vi "drag Markers.vi"(5 "Marker Options":T3={"Color"=16723218, "pen"={"Width"=2, "Style"=enum."Solid"}, "font"={"Font Name"="Arial", "Size"=16, "Strikeout?"=FALSE, "Italic?"=FALSE, "Underline?"=FALSE, "Outline?"=FALSE, "Shadow?"=FALSE, "Bold?"=FALSE, "FontColor"=0}, "caption"=""}, 7 "Type":T2, 10 "Coords":T4, 11 "Plot Area Bounds":T1) -> (3 "new picture":picture)   [LabVIEW 2019]
doc: "Draw notes overlayed on the grph using picture control elements in the graph. This draws a line at the mouse location."
uses:
  <vilib>/Utility/miscctls.llb/LVPoint32TypeDef.ctl
  controls/MarkerOptions.ctl
  controls/markerType.ctl
  <vilib>/Utility/miscctls.llb/LVRectTypeDef.ctl
panel:
  in  "picture":picture
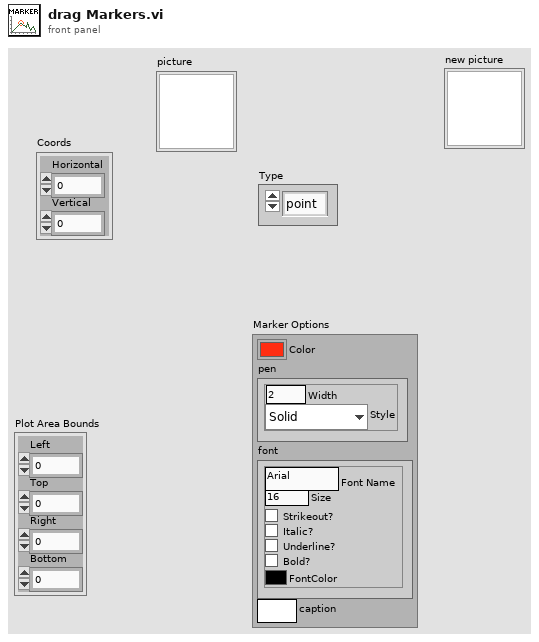
[diagram p1: front panel]
types:
  T1 = typedef "LVRectTypeDef.ctl" = cluster{"Left":i16, "Top":i16, "Right":i16, "Bottom":i16}
  T2 = typedef "markerType.ctl" = enum16{"point", "arrow", "horiz", "vert", "vert range", "horiz range", "box"}
  T3 = typedef "MarkerOptions.ctl" = cluster{"Color":u32, "pen":cluster{"Width":u16, "Style":enum32{"Solid", "Dash", "Dot", "DashDot", "DashDotDot"}}, "font":cluster{"Font Name":string, "Size":i16, "Strikeout?":bool, "Italic?":bool, "Underline?":bool, "Outline?":bool, "Shadow?":bool, "Bold?":bool, "FontColor":u32}, "caption":string}
  T4 = typedef "LVPoint32TypeDef.ctl" = cluster{"Horizontal":i32, "Vertical":i32}
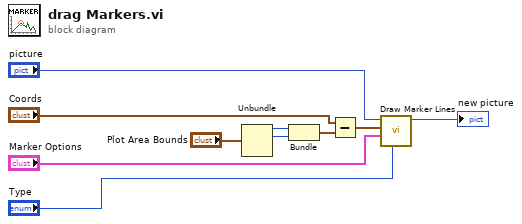
[diagram p0: block diagram]
diagram:
  n1 = Unbundle("Plot Area Bounds") -> ("Left"=w4:i16, "Top"=w5:i16)  [unwired: 2 out]
  n2 = Bundle("Left"=w4, "Top"=w5) -> (w3:cluster{"Left":i16, "Top":i16})  [unwired: 1 in]
  n3 = Subtract(x="Coords", y=w3) -> (x-y=w2:T4)
  n4 = call "Draw Marker Lines.vi"("Type"="Type", "Marker Options"="Marker Options", "position"=w2, "picture"="picture") -> ("new picture"=→"new picture":picture)  [unwired: 7 in]
